vi "Find_VNA_MeasParam_Index.vi"(10 "Instrument Session":string, 11 "VNAs Measurement Parameters":T1) -> (3 "Index":i32)   [LabVIEW 2013]
uses:
  VNAs Measurement Parameters.ctl
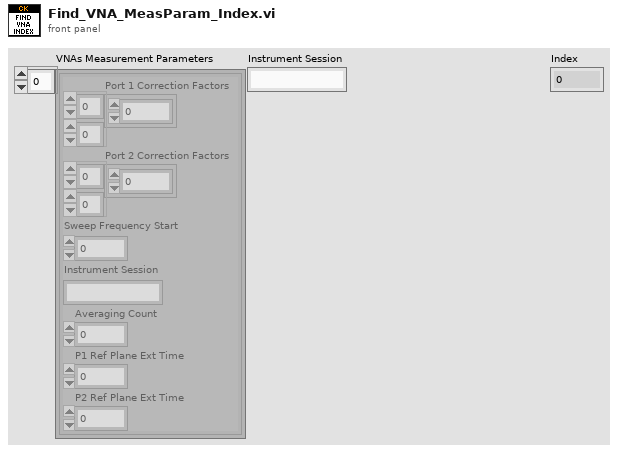
[diagram p1: front panel]
types:
  T1 = typedef "VNAs Measurement Parameters.ctl" = cluster{"Port 1 Correction Factors":cdb[][], "Port 2 Correction Factors":cdb[][], "Sweep Frequency Start":dbl, "Instrument Session":string, "Averaging Count":i32, "P1 Ref Plane Ext Time":dbl, "P2 Ref Plane Ext Time":dbl}[]
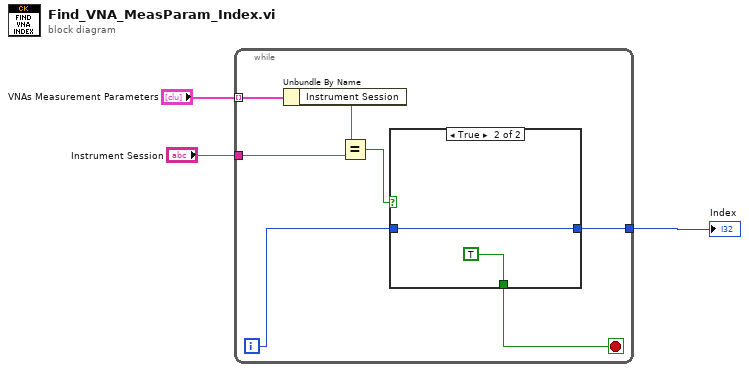
[diagram p0: block diagram]
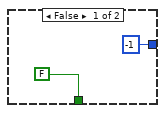
[diagram p2: hidden frame]
diagram:
  n1 = while {
    tunnel: "VNAs Measurement Parameters" -> [w10] mode=indexing
    tunnel: "Instrument Session" -> [w8]
    tunnel: [w4] -> w1
    i -> [w5]
    stop <- w6 stop-if-true
    n2 = Unbundle By Name(w10) -> ("Instrument Session"=w9:string)
    n3 = Equal?(x=w9, y=w8) -> (x = y?=w7:bool)
    n4 = case shown="True" w7 {
      tunnel: [FALSE TRUE] -> w6
      tunnel: w5 -> [_ w13]
      tunnel: [-1 w13] -> w4
      frame False {
      }
      frame True {
      }
    }
  }
  "Index" <- w1
